vi "Model Initial Values - Main On Delete Action.vi"(6 "All deleted Refs":T1[](array[typedef]) format="%.0x", 8 "error in (no error)":errorcluster, 11 "Item Ref in":T1 format="%.0x") -> (0 "error out":errorcluster, 3 "Item Ref out":T1 format="%.0x")   [LabVIEW 2011, in "Model Initial Values Custom Device.lvlib"]
uses:
  Model Initial Values Custom Device.lvlib
  <vilib>/NI Veristand/Custom Device API/Custom Device Item Ref.ctl
  <vilib>/NI Veristand/Custom Device API/Custom Device API.lvlib
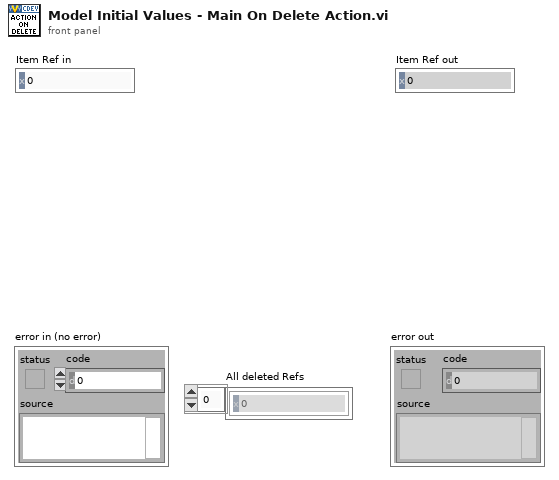
[diagram p1: front panel]
types:
  T1 = typedef "Custom Device API.lvlib/Custom Device Item Ref.ctl" = u64
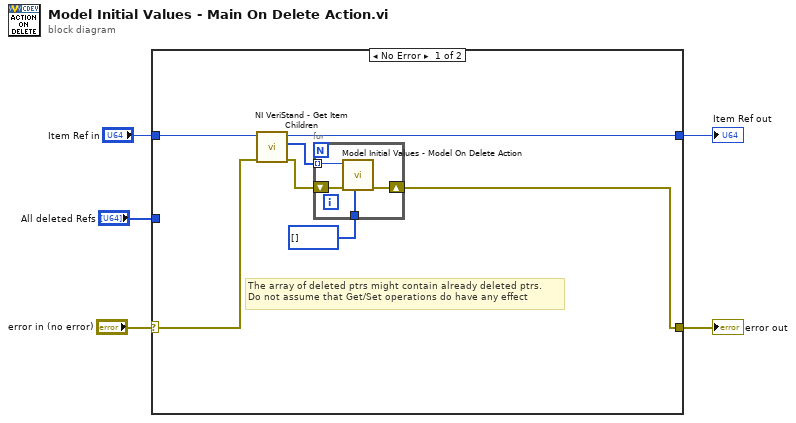
[diagram p0: block diagram]
diagram:
  n1 = case shown="No Error" "error in (no error)" {
    selector: "error in (no error)" -> [w7 w18]
    tunnel: [w6 w18] -> w4
    tunnel: "Item Ref in" -> [w12 w17]
    tunnel: [w11 w17] -> w2
    tunnel: "All deleted Refs" -> [_ _]
    frame No Error {
      # "The array of deleted ptrs might contain already deleted ptrs.\nDo not assume that Get/Set operations do have any effect"
      n2 = call <vilib>:"NI VeriStand - Get Item Children.vi"("error in (no error)"=w7, "Item Ref in"=w12) -> ("error out"=w8:errorcluster, "Child Refs"=w10:T1[], "Item Ref out"=w11:T1)  [unwired: 6 in, 1 out]
      n3 = for {
        shift-right: [w16] -> w6
        shift-left: w8 -> [w15]
        tunnel: w10 -> [w14] mode=indexing
        tunnel: T1[] [] ("All deleted Refs") -> [w13]
        n4 = call "Model Initial Values - Model On Delete Action.vi"("All deleted Refs"=w13, "error in (no error)"=w15, "Item Ref in"=w14) -> ("error out"=w16:errorcluster)  [unwired: 7 in, 1 out]
      }
    }
    frame Error {
    }
  }
  "error out" <- w4
  "Item Ref out" <- w2
